vi "Logging Tree Update Time.vi"(2 "Time":dbl=-1.0, 3 "TreeRef":refnum<vi>) -> (1 "TreeRef":refnum<vi>)   [LabVIEW 2012]
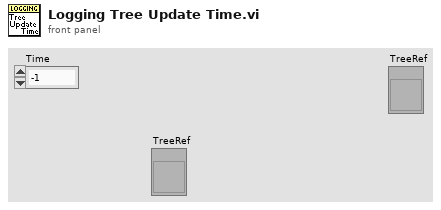
[diagram p1: front panel]
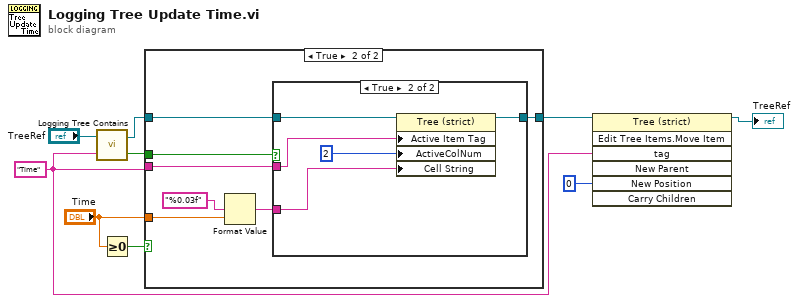
[diagram p0: block diagram]
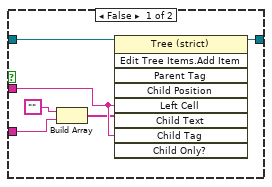
[diagram p3: hidden frame]
diagram:
  w6 = "Time" ("Name")
  n1 = call "Logging Tree Contains.vi"("Name"=w6, "TreeRef"="TreeRef") -> ("Contained"=w9:bool, "TreeRef"=w3:refnum<vi>)
  n2 = Greater Or Equal To 0?(x="Time") -> (x >= 0?=w2:bool)
  n3 = case shown="True" w2 {
    tunnel: w9 -> [_ w17]
    tunnel: w3 -> [w10 w16]
    tunnel: "Time" -> [_ w14]
    tunnel: [w10 w12] -> w7
    tunnel: w6 -> [_ w11]
    frame False {
    }
    frame True {
      n4 = Format Value(format string="%0.03f", value (0)=w14) -> (output string=w13:string)  [unwired: 1 in]
      n5 = case shown="True" w17 {
        tunnel: w11 -> [w22 w27]
        tunnel: w16 -> [w23 w26]
        tunnel: [w21 w25] -> w12
        tunnel: w13 -> [w20 w24]
        frame False {
          n6 = Build Array("", w20) -> (w19:string[])
          n7 = invoke class="Tree (strict)" method="Edit Tree Items.Add Item"(reference=w23, "Left Cell"=w22, "Child Text"=w19, "Child Tag"=w22) -> (reference out=w21:refnum<vi>)  [unwired: 5 in, 8 out]
        }
        frame True {
          n8 = property class="Tree (strict)"(reference=w26, "Active Item Tag"=w27, "ActiveColNum"=2 ("Active Cell:Active Column Number"), "Cell String"=w24) -> (reference out=w25:refnum<vi>)  [unwired: 1 in, 1 out]
        }
      }
    }
  }
  n9 = invoke class="Tree (strict)" method="Edit Tree Items.Move Item"(reference=w7, "tag"=w6, "New Position"=0) -> (reference out=→"TreeRef":refnum<vi>)  [unwired: 4 in, 6 out]
